vi "PH_Powermeter_BaseClass.set GUI Refs.vi"(0 "VI in":refnum<vi>, 1 "Class":string, 2 "Status GUI Reference":refnum<vi>, 3 "Powermeter Base Class GUI References":T1, 4 "PSDB Status GUI Reference":refnum<vi>, 5 "error in (no error)":errorcluster) -> (14 "VI out":refnum<vi>, 19 "error out":errorcluster)   [LabVIEW 2014, in "PH_Powermeter_BaseClass.lvlib"]
uses:
  PH_Powermeter_BaseClass.lvlib
  PH_Powermeter_BaseClass.GUI Refs.ctl
  PH_Powermeter_BaseClass.Head Attributes.ctl
  PH_Powermeter_BaseClass.Energy.ctl
  PH_Powermeter_BaseClass.Connection.ctl
  PH_Powermeter_BaseClass.State.ctl
  PH_gentec_BaseClass.Head Settings.ctl
  PH_PSDBWriter/PH_PSDBWriter.lvlib
  PH_StatusHandler/PH_StatusHandler.lvlib
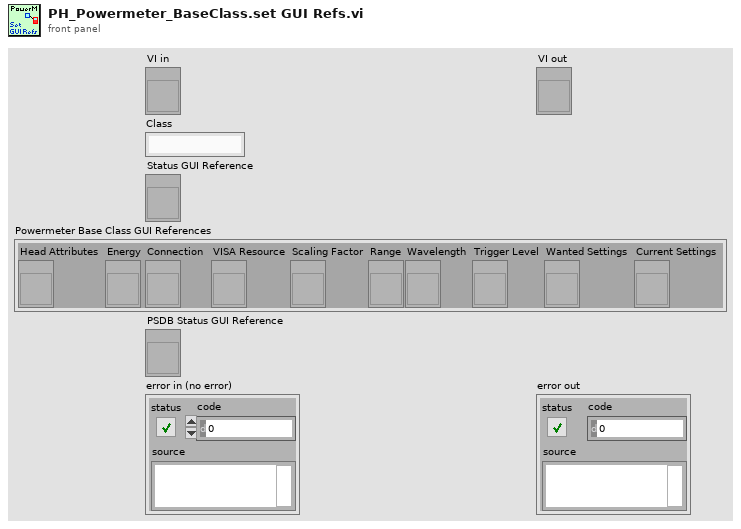
[diagram p1: front panel]
types:
  T1 = typedef "PH_Powermeter_BaseClass.lvlib/PH_Powermeter_BaseClass.GUI Refs.ctl" = cluster{"Head Attributes":refnum<vi>, "Energy":refnum<vi>, "Connection":refnum<vi>, "VISA Resource":refnum<vi>, "Scaling Factor":refnum<vi>, "Range":refnum<vi>, "Wavelength":refnum<vi>, "Trigger Level":refnum<vi>, "Wanted Settings":refnum<vi>, "Current Settings":refnum<vi>}
  T2 = typedef "PH_Powermeter_BaseClass.lvlib/PH_Powermeter_BaseClass.i attribute.ctl" = cluster{"GUI References":T1, "Connection":T3, "Head Attributes":T5, "VISA resource":refnum<visa-resource-name>, "Energy":T6, "Service ID Energy":i32, "Wanted Settings":T7, "Current Settings":T7}
  T3 = typedef "PH_Powermeter_BaseClass.lvlib/PH_Powermeter_BaseClass.Connection.ctl" = cluster{"failed checks":i8, "Timeout":bool, "Data read":string, "Failure":bool, "Error":bool, "State":T4}
  T4 = typedef "PH_Powermeter_BaseClass.lvlib/PH_Powermeter_BaseClass.State.ctl" = enum32{"off", "operating", "opened", "checked", "connected", "Sets to change", "running"}
  T5 = typedef "PH_Powermeter_BaseClass.lvlib/PH_Powermeter_BaseClass.Head Attributes.ctl" = cluster{"Instrument Type":string, "Head Version":string, "Head Name":string, "Serial Number":string, "Firmware":string, "Sensor Type":string, "MinimumRange":u32, "Maximum Range":u32, "Min Wavelength":i32, "Max Wavelength":i32}
  T6 = typedef "PH_Powermeter_BaseClass.lvlib/PH_Powermeter_BaseClass.Energy.ctl" = cluster{"current Value":dbl, "unscaled":dbl, "Scaling Factor":dbl}
  T7 = typedef "PH_Powermeter_BaseClass.lvlib/PH_gentec_BaseClass.Head Settings.ctl" = cluster{"Trigger Level":dbl, "Wavelength":u32, "Range":u32}
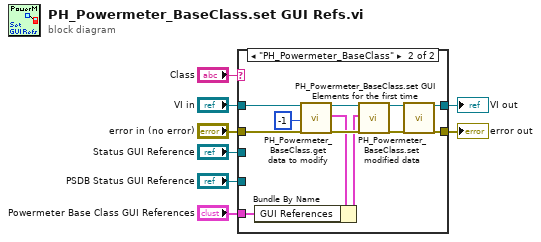
[diagram p0: block diagram]
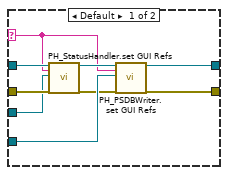
[diagram p2: hidden frame]
diagram:
  n1 = case shown="\"PH_Powermeter_BaseClass\"" "Class" {
    selector: "Class" -> [w10 _]
    tunnel: "VI in" -> [w12 w25]
    tunnel: "error in (no error)" -> [w17 w24]
    tunnel: [w16 w21] -> w6
    tunnel: [w15 w20] -> w7
    tunnel: "Status GUI Reference" -> [w9 _]
    tunnel: "PSDB Status GUI Reference" -> [w14 _]
    tunnel: "Powermeter Base Class GUI References" -> [_ w18]
    frame Default {
      n2 = call "PH_StatusHandler.set GUI Refs.vi"("i ref in"=w12, "Class"=w10, "GUI Ref"=w9, "error in (no error)"=w17) -> ("i ref out"=w11:refnum<vi>, "error out"=w13:errorcluster)  [unwired: 14 in]
      n3 = call "PH_PSDBWriter.set GUI Refs.vi"("i ref in"=w11, "Class"=w10, "Ref PSDB Status"=w14, "error in"=w13) -> ("i ref out"=w16:refnum<vi>, "error out"=w15:errorcluster)  [unwired: 14 in]
    }
    frame "PH_Powermeter_BaseClass" {
      n4 = call "PH_Powermeter_BaseClass.get data to modify.vi"("i ref in"=w25, "ms timeout (10000)"=-1, "error in (no error)"=w24) -> ("i ref out"=w29:refnum<vi>, "i attribute"=w26:T2, "error out"=w28:errorcluster)  [unwired: 13 in, 1 out]
      n5 = Bundle By Name(cluster=w26, "GUI References"=w18) -> (w19:T2)
      n6 = call "PH_Powermeter_BaseClass.set modified data.vi"("i ref in"=w29, "i attribute"=w19, "error in (no error)"=w28) -> ("i ref out"=w22:refnum<vi>, "error out"=w23:errorcluster)  [unwired: 15 in]
      n7 = call "PH_Powermeter_BaseClass.set GUI Elements for the first time.vi"("i ref in"=w22, "error in"=w23) -> ("i ref out"=w21:refnum<vi>, "error out"=w20:errorcluster)  [unwired: 16 in]
    }
  }
  "error out" <- w7
  "VI out" <- w6
